vi "Get Aircraft System Status.vi"(8 "Error In":errorcluster, 11 "Aircraft ID":u8) -> (0 "Error Out":errorcluster, 3 "System Status Out":T1 {"Communication Drop Rate (%)" scale=0.0..100.0; "Battery Remaining (%)" scale=0.0..100.0; "CPU Load (%)" scale=0.0..100.0})   [LabVIEW 2014]
uses:
  Controls/Aircraft Sensor Status Data.ctl
  GUI Design/Indicators/Sensor Status LED CLuster.ctl
  GUI Design/Indicators/Status LED.ctl
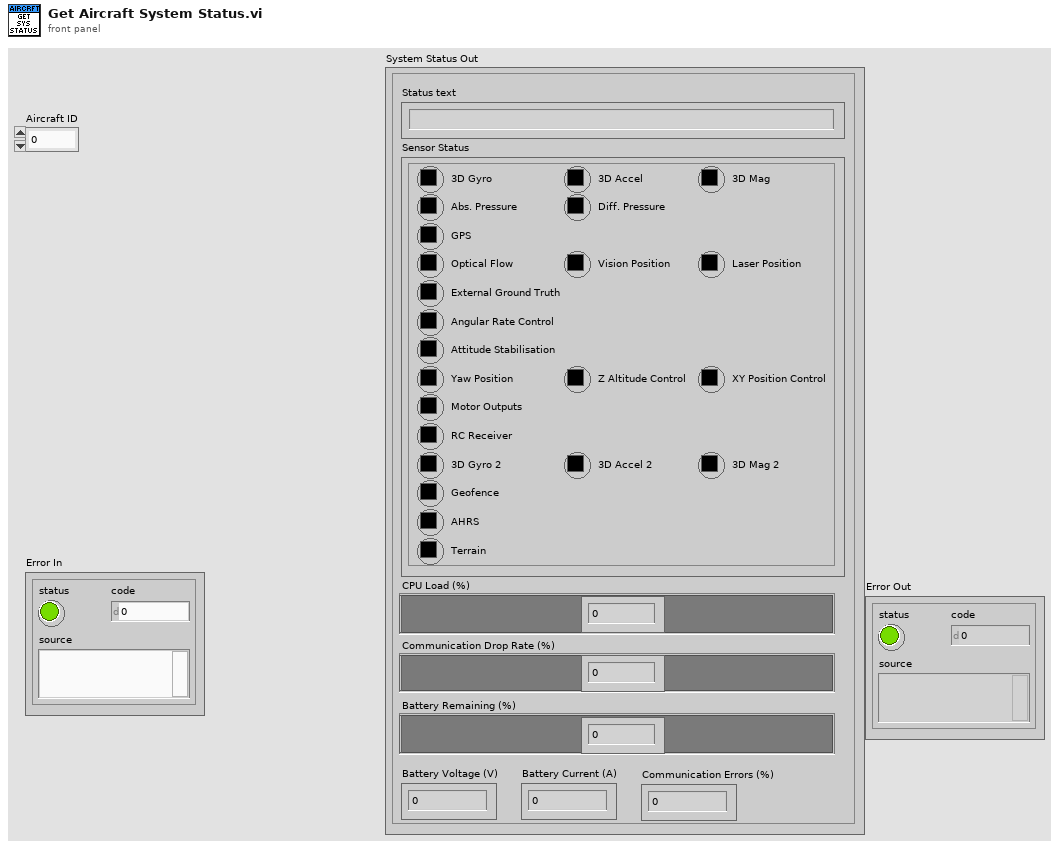
[diagram p1: front panel]
types:
  T1 = typedef "Aircraft Sensor Status Data.ctl" = cluster{"Sensor Status":T2, "CPU Load (%)":dbl, "Battery Voltage (V)":dbl, "Battery Current (A)":dbl, "Battery Remaining (%)":dbl, "Communication Drop Rate (%)":dbl, "Communication Errors (%)":dbl, "Status text":string}
  T2 = typedef "Sensor Status LED CLuster.ctl" = cluster{"3D Gyro":u32, "3D Accel":u32, "3D Mag":u32, "Abs. Pressure":u32, "Diff. Pressure":u32, "GPS":T3, "Optical Flow":u32, "Vision Position":u32, "Laser Position":u32, "External Ground Truth":u32, "Angular Rate Control":u32, "Attitude Stabilisation":u32, "Yaw Position":u32, "Z Altitude Control":u32, "XY Position Control":u32, "Motor Outputs":u32, "RC Receiver":u32, "3D Gyro 2":u32, "3D Accel 2":u32, "3D Mag 2":u32, "Geofence":u32, "AHRS":u32, "Terrain":u32}
  T3 = typedef "Status LED.ctl" = u32
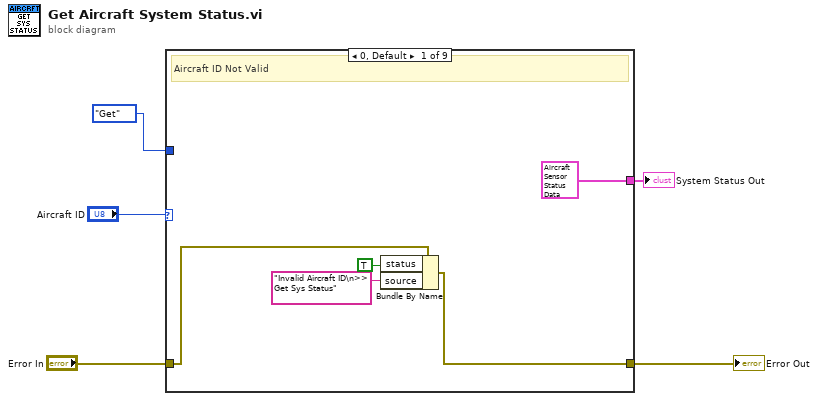
[diagram p0: block diagram]
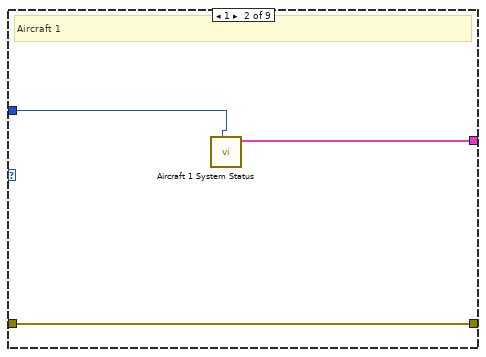
[diagram p2: hidden frame]
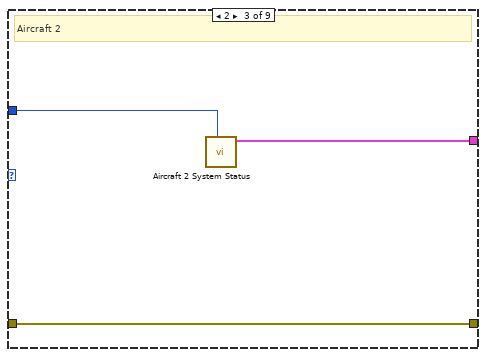
[diagram p3: hidden frame]
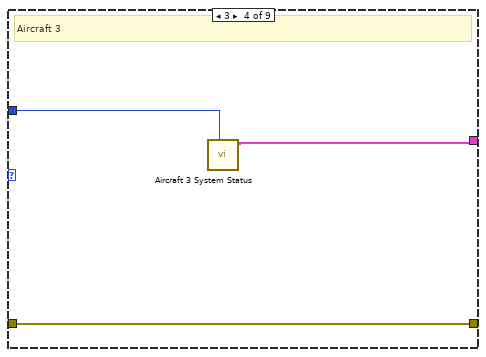
[diagram p4: hidden frame]
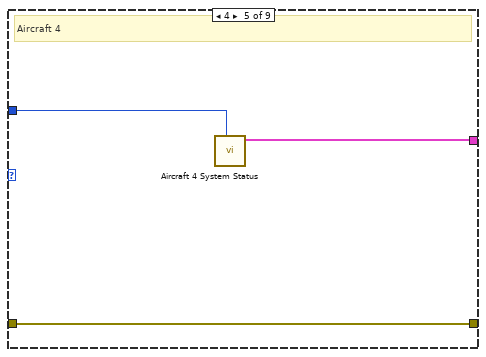
[diagram p5: hidden frame]
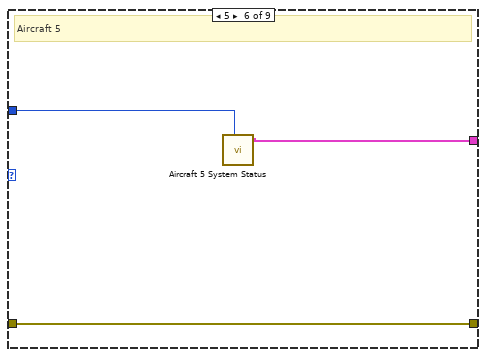
[diagram p6: hidden frame]
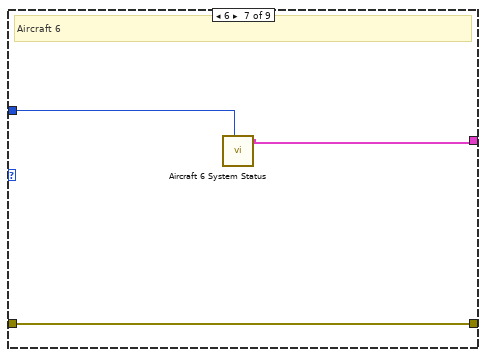
[diagram p7: hidden frame]
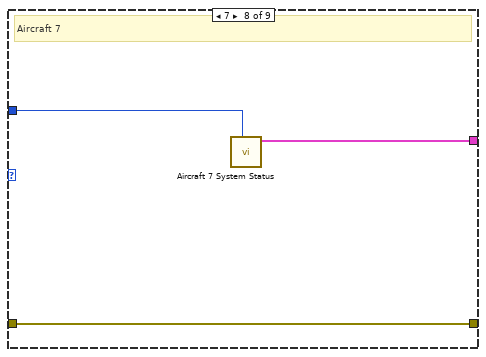
[diagram p8: hidden frame]
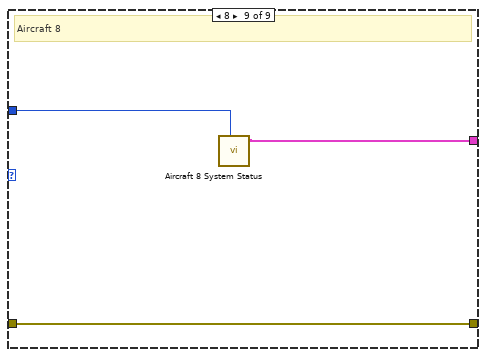
[diagram p9: hidden frame]
diagram:
  n1 = case shown="0, Default" "Aircraft ID" {
    tunnel: [T1 {"Sensor Status"={"3D Gyro"=0, "3D Accel"=0, "3D Mag"=0, "Abs. Pressure"=0, "Diff. Pressure"=0, "GPS"=0, "Optical Flow"=0, "Vision Position"=0, "Laser Position"=0, "External Ground Truth"=0, "Angular Rate Control"=0, "Attitude Stabilisation"=0, "Yaw Position"=0, "Z Altitude Control"=0, "XY Position Control"=0, "Motor Outputs"=0, "RC Receiver"=0, "3D Gyro 2"=0, "3D Accel 2"=0, "3D Mag 2"=0, "Geofence"=0, "AHRS"=0, "Terrain"=0}, "CPU Load (%)"=0.0, "Battery Voltage (V)"=0.0, "Battery Current (A)"=0.0, "Battery Remaining (%)"=0.0, "Communication Drop Rate (%)"=0.0, "Communication Errors (%)"=0.0, "Status text"=""} ("System Status Out") w12 w15 w18 w21 w24 w27 w30 w33] -> w1
    tunnel: [w9 w13 w16 w19 w22 w25 w28 w31 w34] -> w4
    tunnel: "Error In" -> [w10 w13 w16 w19 w22 w25 w28 w31 w34]
    tunnel: enum16{"Get", "Set"}."Get" ("Method") -> [_ w11 w14 w17 w20 w23 w26 w29 w32]
    frame 0, Default {
      # "Aircraft ID Not Valid"
      n2 = Bundle By Name(cluster=w10, "status"=TRUE, "source"="Invalid Aircraft ID\n>> Get Sys Status") -> (w9:errorcluster)
    }
    frame 1 {
      # "Aircraft 1"
      n3 = call "Aircraft 1 System Status.vi"("Method"=w11) -> ("System Status Out"=w12:T1)  [unwired: 10 in]
    }
    frame 2 {
      # "Aircraft 2"
      n4 = call "Aircraft 2 System Status.vi"("Method"=w14) -> ("System Status Out"=w15:T1)  [unwired: 10 in]
    }
    frame 3 {
      # "Aircraft 3"
      n5 = call "Aircraft 3 System Status.vi"("Method"=w17) -> ("System Status Out"=w18:T1)  [unwired: 10 in]
    }
    frame 4 {
      # "Aircraft 4"
      n6 = call "Aircraft 4 System Status.vi"("Method"=w20) -> ("System Status Out"=w21:T1)  [unwired: 10 in]
    }
    frame 5 {
      # "Aircraft 5"
      n7 = call "Aircraft 5 System Status.vi"("Method"=w23) -> ("System Status Out"=w24:T1)  [unwired: 10 in]
    }
    frame 6 {
      # "Aircraft 6"
      n8 = call "Aircraft 6 System Status.vi"("Method"=w26) -> ("System Status Out"=w27:T1)  [unwired: 10 in]
    }
    frame 7 {
      # "Aircraft 7"
      n9 = call "Aircraft 7 System Status.vi"("Method"=w29) -> ("System Status Out"=w30:T1)  [unwired: 10 in]
    }
    frame 8 {
      # "Aircraft 8"
      n10 = call "Aircraft 8 System Status.vi"("Method"=w32) -> ("System Status Out"=w33:T1)  [unwired: 10 in]
    }
  }
  "Error Out" <- w4
  "System Status Out" <- w1
